vi "Reply.vi"(8 "error in (no error)":errorcluster, 9 "Result":variant, 10 "request":refnum<class "request.lvclass">, 11 "output_actor in":refnum<class "Output Actor.lvclass">) -> (0 "error out":errorcluster, 3 "output_actor out":refnum<class "Output Actor.lvclass">)   [LabVIEW 2015, in "Output Actor.lvclass"]
uses:
  Output Actor.lvclass
  Request/request.lvclass
  Output Actor.lvclass/Output Actor.ctl
  Output/Output.lvclass
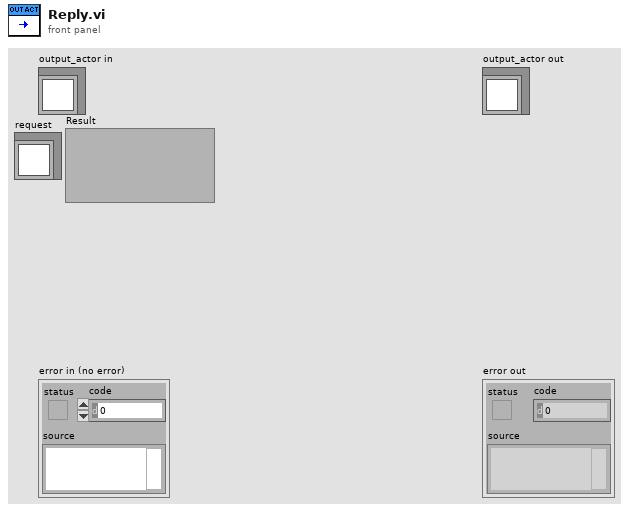
[diagram p1: front panel]
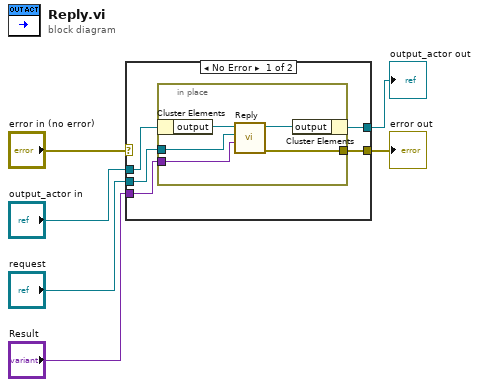
[diagram p0: block diagram]
diagram:
  n1 = case shown="No Error" "error in (no error)" {
    selector: "error in (no error)" -> [_ w18]
    tunnel: [w7 w18] -> w5
    tunnel: [w8 w17] -> w3
    tunnel: "output_actor in" -> [w11 w17]
    tunnel: "request" -> [w10 _]
    tunnel: "Result" -> [w9 _]
    frame No Error {
      n2 = in-place {
        in-place-border: [w14] -> w7
        in-place-border: w10 -> [w13]
        in-place-border: w9 -> [w12]
        n3 = in-place-cluster #1(w11) -> ("output"=w16:refnum<class "Output.lvclass">)
        n4 = call "Reply.vi"("parameter"=w12, "request"=w13, "output in"=w16) -> ("error out"=w14:errorcluster, "output out"=w15:refnum<class "Output.lvclass">)  [unwired: 7 in]
        n5 = in-place-cluster #1("output"=w15) -> (w8:refnum<class "Output Actor.lvclass">)
      }
    }
    frame Error {
    }
  }
  "error out" <- w5
  "output_actor out" <- w3
